vi "Q8381 Graph Data Convert.vi"(1 "Input Data":T1 {"Y Axis Data" format="%.5e"; "X Axis Data" format="%.5e"}) -> (0 "Output Data":T1 {"Y Axis Data" format="%.5f"; "X Axis Data" format="%.5f"})   [LabVIEW 2017]
doc: "Multiply first array elements by one million and leave second array elements as it is."
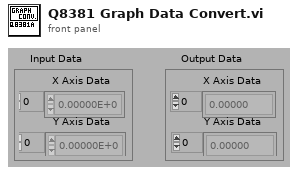
[diagram p1: front panel]
types:
  T1 = cluster{"X Axis Data":dbl[], "Y Axis Data":dbl[]}
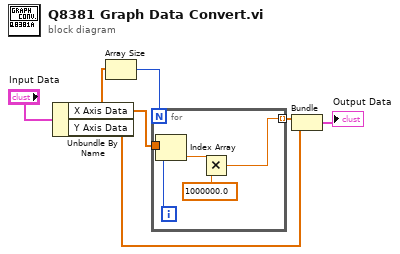
[diagram p0: block diagram]
diagram:
  n1 = Unbundle By Name("Input Data") -> ("X Axis Data"=w4:dbl[], "Y Axis Data"=w2:dbl[])
  n2 = Array Size(array=w4) -> (size(s)=w5:i32)
  n3 = for {
    N: w5 -> [_]
    tunnel: w4 -> [w10]
    tunnel: [w7] -> w3 mode=indexing
    i -> [w11]
    n4 = Index Array(array=w10, index=w11) -> (element=w9:dbl)
    n5 = Multiply(x=w9, y=1000000.0) -> (x*y=w7:dbl)
  }
  n6 = Bundle(w3, "Y Axis Data"=w2) -> (→"Output Data":cluster{dbl[], "Y Axis Data":dbl[]})  [unwired: 1 in]
